vi "_word.GetBookmarkByName.vi"(8 "error in (no error)":errorcluster, 10 "String":string, 11 "Document":refnum<k7>) -> (0 "error out":errorcluster, 1 "found":bool, 2 "bookmark":refnum<k7>, 3 "Document(dup)":refnum<k7>)   [LabVIEW 2018, in "WordReportGeneration.lvlib"]
uses:
  WordReportGeneration.lvlib
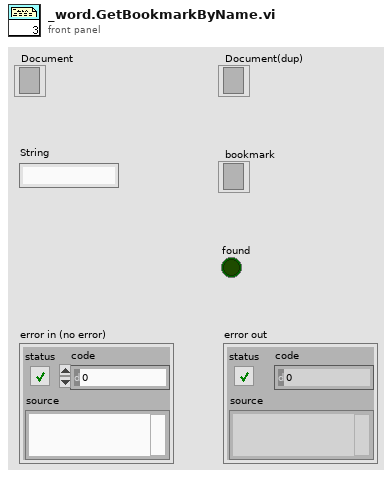
[diagram p1: front panel]
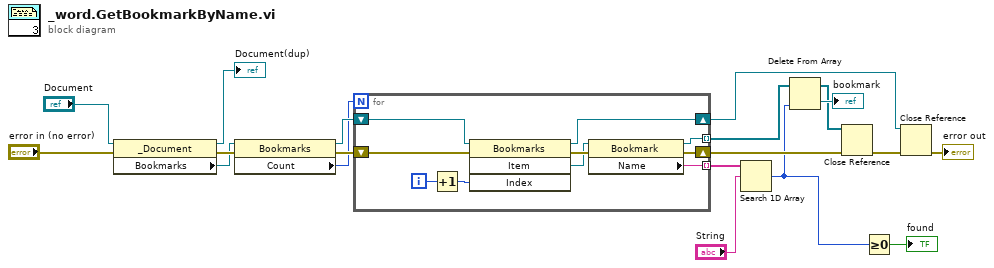
[diagram p0: block diagram]
diagram:
  n1 = property class="_Document"(reference="Document", error in="error in (no error)") -> (reference out=→"Document(dup)":refnum<k7>, error out=w17:errorcluster, "Bookmarks"=w16:refnum<k7>)
  n2 = property class="Bookmarks"(reference=w16, error in=w17) -> (reference out=w5:refnum<k7>, error out=w7:errorcluster, "Count"=w3:i32)
  n3 = for {
    N: w3 -> [_]
    tunnel: [w25] -> w13 mode=indexing
    shift-right: [w21] -> w8
    shift-left: w7 -> [w24]
    shift-right: [w22] -> w4
    shift-left: w5 -> [w23]
    tunnel: [w20] -> w11 mode=indexing
    i -> [w28]
    n4 = Increment(x=w28) -> (x+1=w27:i32)
    n5 = invoke class="Bookmarks" method="Item"(reference=w23, error in=w24, "Index"=w27) -> (reference out=w22:refnum<k7>, error out=w29:errorcluster, "Item"=w26:refnum<k7>)  [unwired: 1 in, 1 out]
    n6 = property class="Bookmark"(reference=w26, error in=w29) -> (reference out=w20:refnum<k7>, error out=w21:errorcluster, "Name"=w25:string)
  }
  n7 = Search 1D Array(1D array=w13, element="String") -> (index of element=w2:i32)  [unwired: 1 in]
  n8 = Delete From Array(array=w11, index=w2) -> (deleted portion=→"bookmark":refnum<k7>, array with subset deleted=w9:refnum<k7>[])  [unwired: 1 in]
  n9 = Close Reference(reference=w9, error in (no error)=w8) -> (error out=w6:errorcluster)
  n10 = Greater Or Equal To 0?(x=w2) -> (x >= 0?=→"found":bool)
  n11 = Close Reference(reference=w4, error in (no error)=w6) -> (error out=→"error out":errorcluster)
